vi "Gear Up.vi"(3 "Step":i32, 5 "Startup":bool) -> (0 "Completed":bool, 1 "Output":dbl)   [LabVIEW 2016]
uses:
  Command Execution State.ctl
  Rotation/Rotation Globals.vi
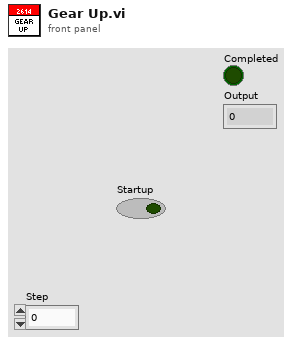
[diagram p1: front panel]
types:
  T1 = typedef "Command Execution State.ctl" = enum16{"Initialize", "Execute", "Finish"}
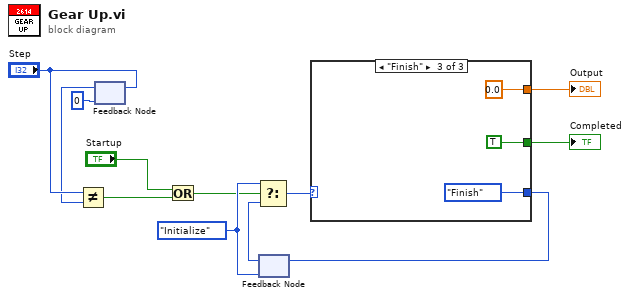
[diagram p0: block diagram]
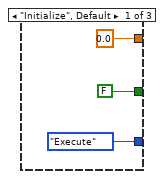
[diagram p2: hidden frame]
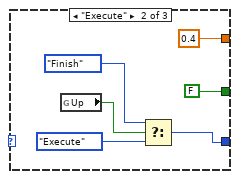
[diagram p3: hidden frame]
diagram:
  w8 = Command_Execution_State."Initialize" ("Play State")
  n1 = feedback #1(0 ("Step")) -> (w4:i32)
  n2 = Not Equal?(x="Step", y=w4) -> (x != y?=w2:bool)
  n3 = feedback-in #1("Step") -> ()
  n4 = Or(x="Startup", y=w2) -> (x .or. y?=w3:bool)
  n5 = feedback #2(w8) -> (w9:T1)
  n6 = Select(t=w8, s=w3, f=w9) -> (s? t:f=w12:T1)
  n7 = case shown="\"Finish\"" w12 {
    tunnel: [Command_Execution_State."Execute" ("Play State") w21 Command_Execution_State."Finish" ("Play State")] -> w10
    tunnel: [FALSE FALSE TRUE] -> w7
    tunnel: [0.0 ("Command") 0.4 ("f") 0.0 ("Command")] -> w6
    frame "Initialize", Default {
    }
    frame "Execute" {
      n8 = global read "Rotation Globals.vi" "Up"() -> (w16:bool)
      n9 = Select(t=Command_Execution_State."Finish" ("Play State"), s=w16, f=Command_Execution_State."Execute" ("Play State")) -> (s? t:f=w21:T1)
    }
    frame "Finish" {
    }
  }
  "Completed" <- w7
  "Output" <- w6
  n10 = feedback-in #2(w10) -> ()
